vi "getCommentFromXmlNative.vi"(8 "error in (no error)":errorcluster, 10 "eventXML":refnum<k20>, 11 "ScriptEvent in":refnum<class "ScriptEvent.lvclass">) -> (0 "error out":errorcluster, 2 "eventXML out":refnum<k20>, 3 "ScriptEvent out":refnum<class "ScriptEvent.lvclass">)   [LabVIEW 2011, in "Tools.lvlib" / "Scripting.lvlib" / "ScriptEvent.lvclass"]
uses:
  ScriptEvent.lvclass
  <vilib>/xml/Close Reference(Node).vi
  <vilib>/xml/NI_XML.lvlib
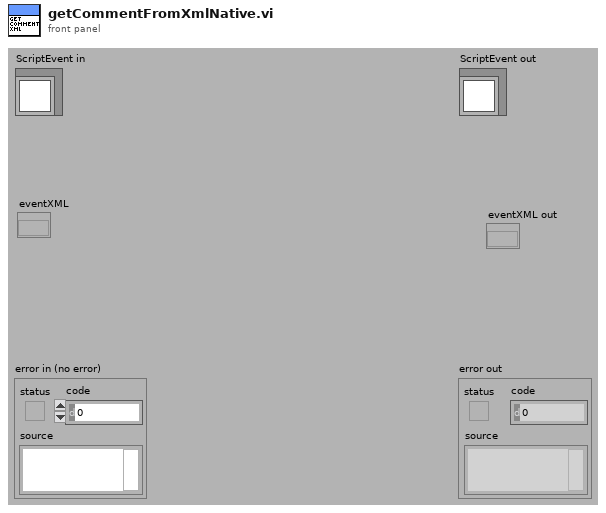
[diagram p1: front panel]
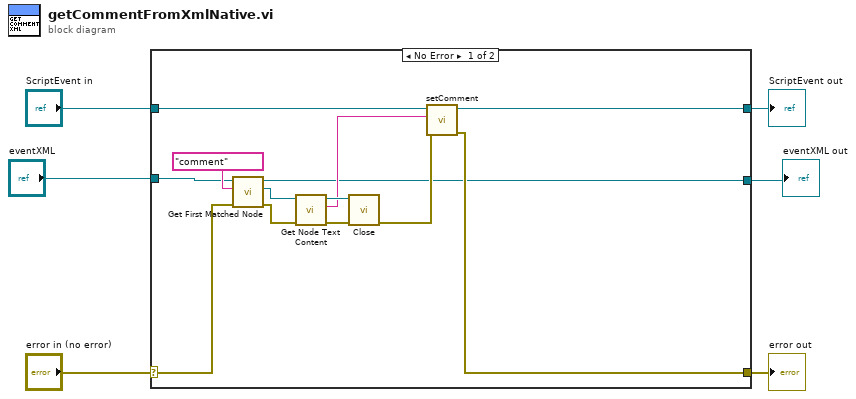
[diagram p0: block diagram]
diagram:
  n1 = case shown="No Error" "error in (no error)" {
    selector: "error in (no error)" -> [w8 w21]
    tunnel: [w9 w21] -> w5
    tunnel: [w13 w20] -> w3
    tunnel: "ScriptEvent in" -> [w12 w20]
    tunnel: "eventXML" -> [w14 _]
    tunnel: [w7 _] -> w1
    frame No Error {
      n2 = call <vilib>:"Get First Matched Node.vi"("error in (no error)"=w8, "XPath expression"="comment", "node in"=w14) -> ("error out"=w18:errorcluster, "node result"=w17:refnum<k20>, "node out"=w7:refnum<k20>)  [unwired: 6 in]
      n3 = call <vilib>:"Get Node Text Content.vi"("error in (no error)"=w18, "node in"=w17) -> ("error out"=w16:errorcluster, "node text"=w10:string, "node out"=w15:refnum<k20>)  [unwired: 7 in]
      n4 = call-poly <vilib>:"Close.vi"("error in (no error)"=w16, "node"=w15) -> ("error out"=w11:errorcluster)  [unwired: 7 in]
      n5 = call-dynamic "setComment.vi"("error in (no error)"=w11, "comment"=w10, "ScriptEvent.lvclass in"=w12) -> ("error out"=w9:errorcluster, "ScriptEvent.lvclass out"=w13:refnum<class "ScriptEvent.lvclass">)  [unwired: 7 in]
    }
    frame Error {
    }
  }
  "error out" <- w5
  "ScriptEvent out" <- w3
  "eventXML out" <- w1
